vi "ui-event.vi"() -> ()   [LabVIEW 2013]
panel:
  out "当前时间":timestamp
  in  "时间检查":bool
  out "迭代":i32
  in  "停止":bool
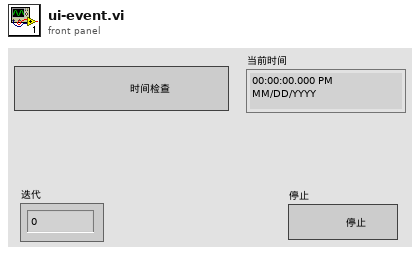
[diagram p1: front panel]
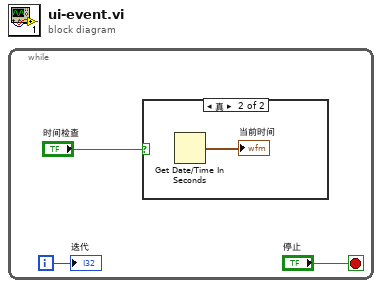
[diagram p0: block diagram]
diagram:
  n1 = while {
    i -> [w2]
    stop <- "停止" stop-if-true
    n2 = case shown="真" "时间检查" {
      frame False {
      }
      frame True {
        n3 = Get Date/Time In Seconds ("获取日期/时间（秒）")() -> (seconds since 1Jan1904=→"当前时间":timestamp)
      }
    }
    "迭代" <- w2
  }
